vi "ProcessPulses_v1k.vi"() -> ()   [LabVIEW 2013]
uses:
  <vilib>/Utility/error.llb/whitespace.ctl
  <vilib>/Analysis/baseanly.llb/Mean (DBL).vi
  <vilib>/Utility/file.llb/Read From Spreadsheet File (DBL).vi
  <vilib>/Utility/file.llb/Read From Spreadsheet File (string).vi
  <vilib>/Analysis/NI_AALBase.lvlib
panel:
  in  "Stop All":bool
  in  "Tab Control":enum32{"Isotope Results", "Summary Table"}(tab)
  in  "AddedToSummary?":bool
  in  "CalculationDone?":bool
  in  "FileLoaded?":bool
  in  "FileSuffix":string=".str.csv"
  in  "AnalysisID":u32 format="%04.0f"
  in  "PulseDataFilesDirectory":path
  in  "FileToLoadExists?":bool
  in  "ExpressLoad":bool
  in  "FileToLoad":path
  in  "MessageOut":string
  out "Cycle Data":dbl[][](array[numeric])
  out "CycleData":string[](array[string])
  out "Pulse Data":dbl[][](array[numeric])
  out "Results array loaded from file:":path
  out "low":dbl format="%.2f"
  out "high":dbl format="%.2f"
  out "width":dbl format="%.2f"
  in  "Confidence Level":dbl=95.0 format="%#.2f"
  in  "Open a saved spreadsheet?":bool
  out "rel mean diff Press vs Ref":dbl format="%.2f"
  out "Ratios, Sam/Ref":dbl[][](array[numeric]) format="%10.2f"
  out "diff MR CH4 vs Ref":dbl format="%.2f"
  in  "Line to clear from array:":i32
  in  "Clear this line?":bool
  out "Results array saved to file:":path
  in  "Save array to spreadsheet? (NOT FUNCTIONAL YET)":bool
  in  "Last Cycle to Use":i32=16
  in  "First Cycle to Use":dbl=1.0
  out "# of Comparisons":i32
  in  "Calculate Now?":bool
  out "Mean and SD Ratios":dbl[][](array[numeric]) format="%10.2f"
  in  "Which Order?":enum16{"No Calculation", "Ref-Sam", "Sam-Ref"}(ring)=enum."Sam-Ref" caption="Calculate using which sam/ref order?"
  out "diff Press vs Ref":dbl format="%.2f"
  in  "Method":T1(ring)
  in  "PulseData":string[](array[string])
  in  "AutoScroll?":bool=TRUE
  out "tStampToAppend":string
  out "SummaryTableTimestamps":string[](array[string]) caption="ISO-8601 Timestamp"
  in  "Save Table to File?":bool
  in  "Clear whole table?":bool
  in  "SummaryTableFilePath":path
  out "FilenameToBeAdded":string
  out "Array to Append":dbl[](array[numeric])
  in  "Line to clear from Summary":i32
  in  "Clear line from Summary?":bool
  out "SummaryTableLineNumber":i32[](array[numeric]) caption="Line #"
  out "SummaryTableFilenames":string[](array[string]) caption="STR Filename"
  out "SummaryTable":string[](array[string])
  out "Summary Table":dbl[][](array[numeric])
  in  "Add to Summary?":bool
  # "EXPRESS Keyboard Shortcuts:   [F1] Increment Filename,  [F2] Load File,  [F3] Calculate,  [F4] Add Results to Summary Table,  [F5] Change focus to Isotope Results Tab"
  # "(zero-indexed)"
  # "(pop up dialog will open)"
  # "(this menu only used for S-R or R-S \ncomparison method)"
  # "(pop up dialog will open)"
  # "Q/Qref - 1"
  # "Q/Qref - 1"
  # "d13, dD, d13D, D13D\nstdev's"
  # "%"
  # "%"
  # "%"
  # "%"
  # "(zero-indexed)"
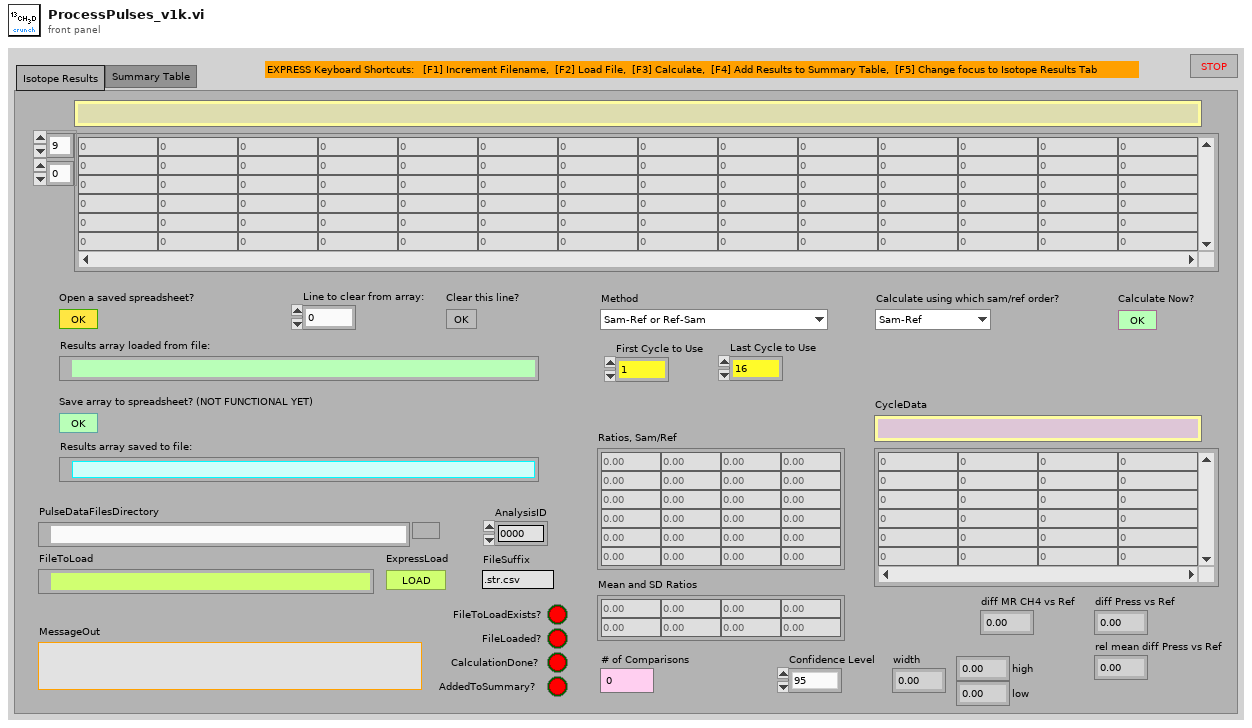
[diagram p1: front panel]
types:
  T1 = enum16{"Sam-Ref or Ref-Sam", "Recycle (Ref-Sam-Ref)"}
  T2 = typedef "whitespace.ctl" = u16
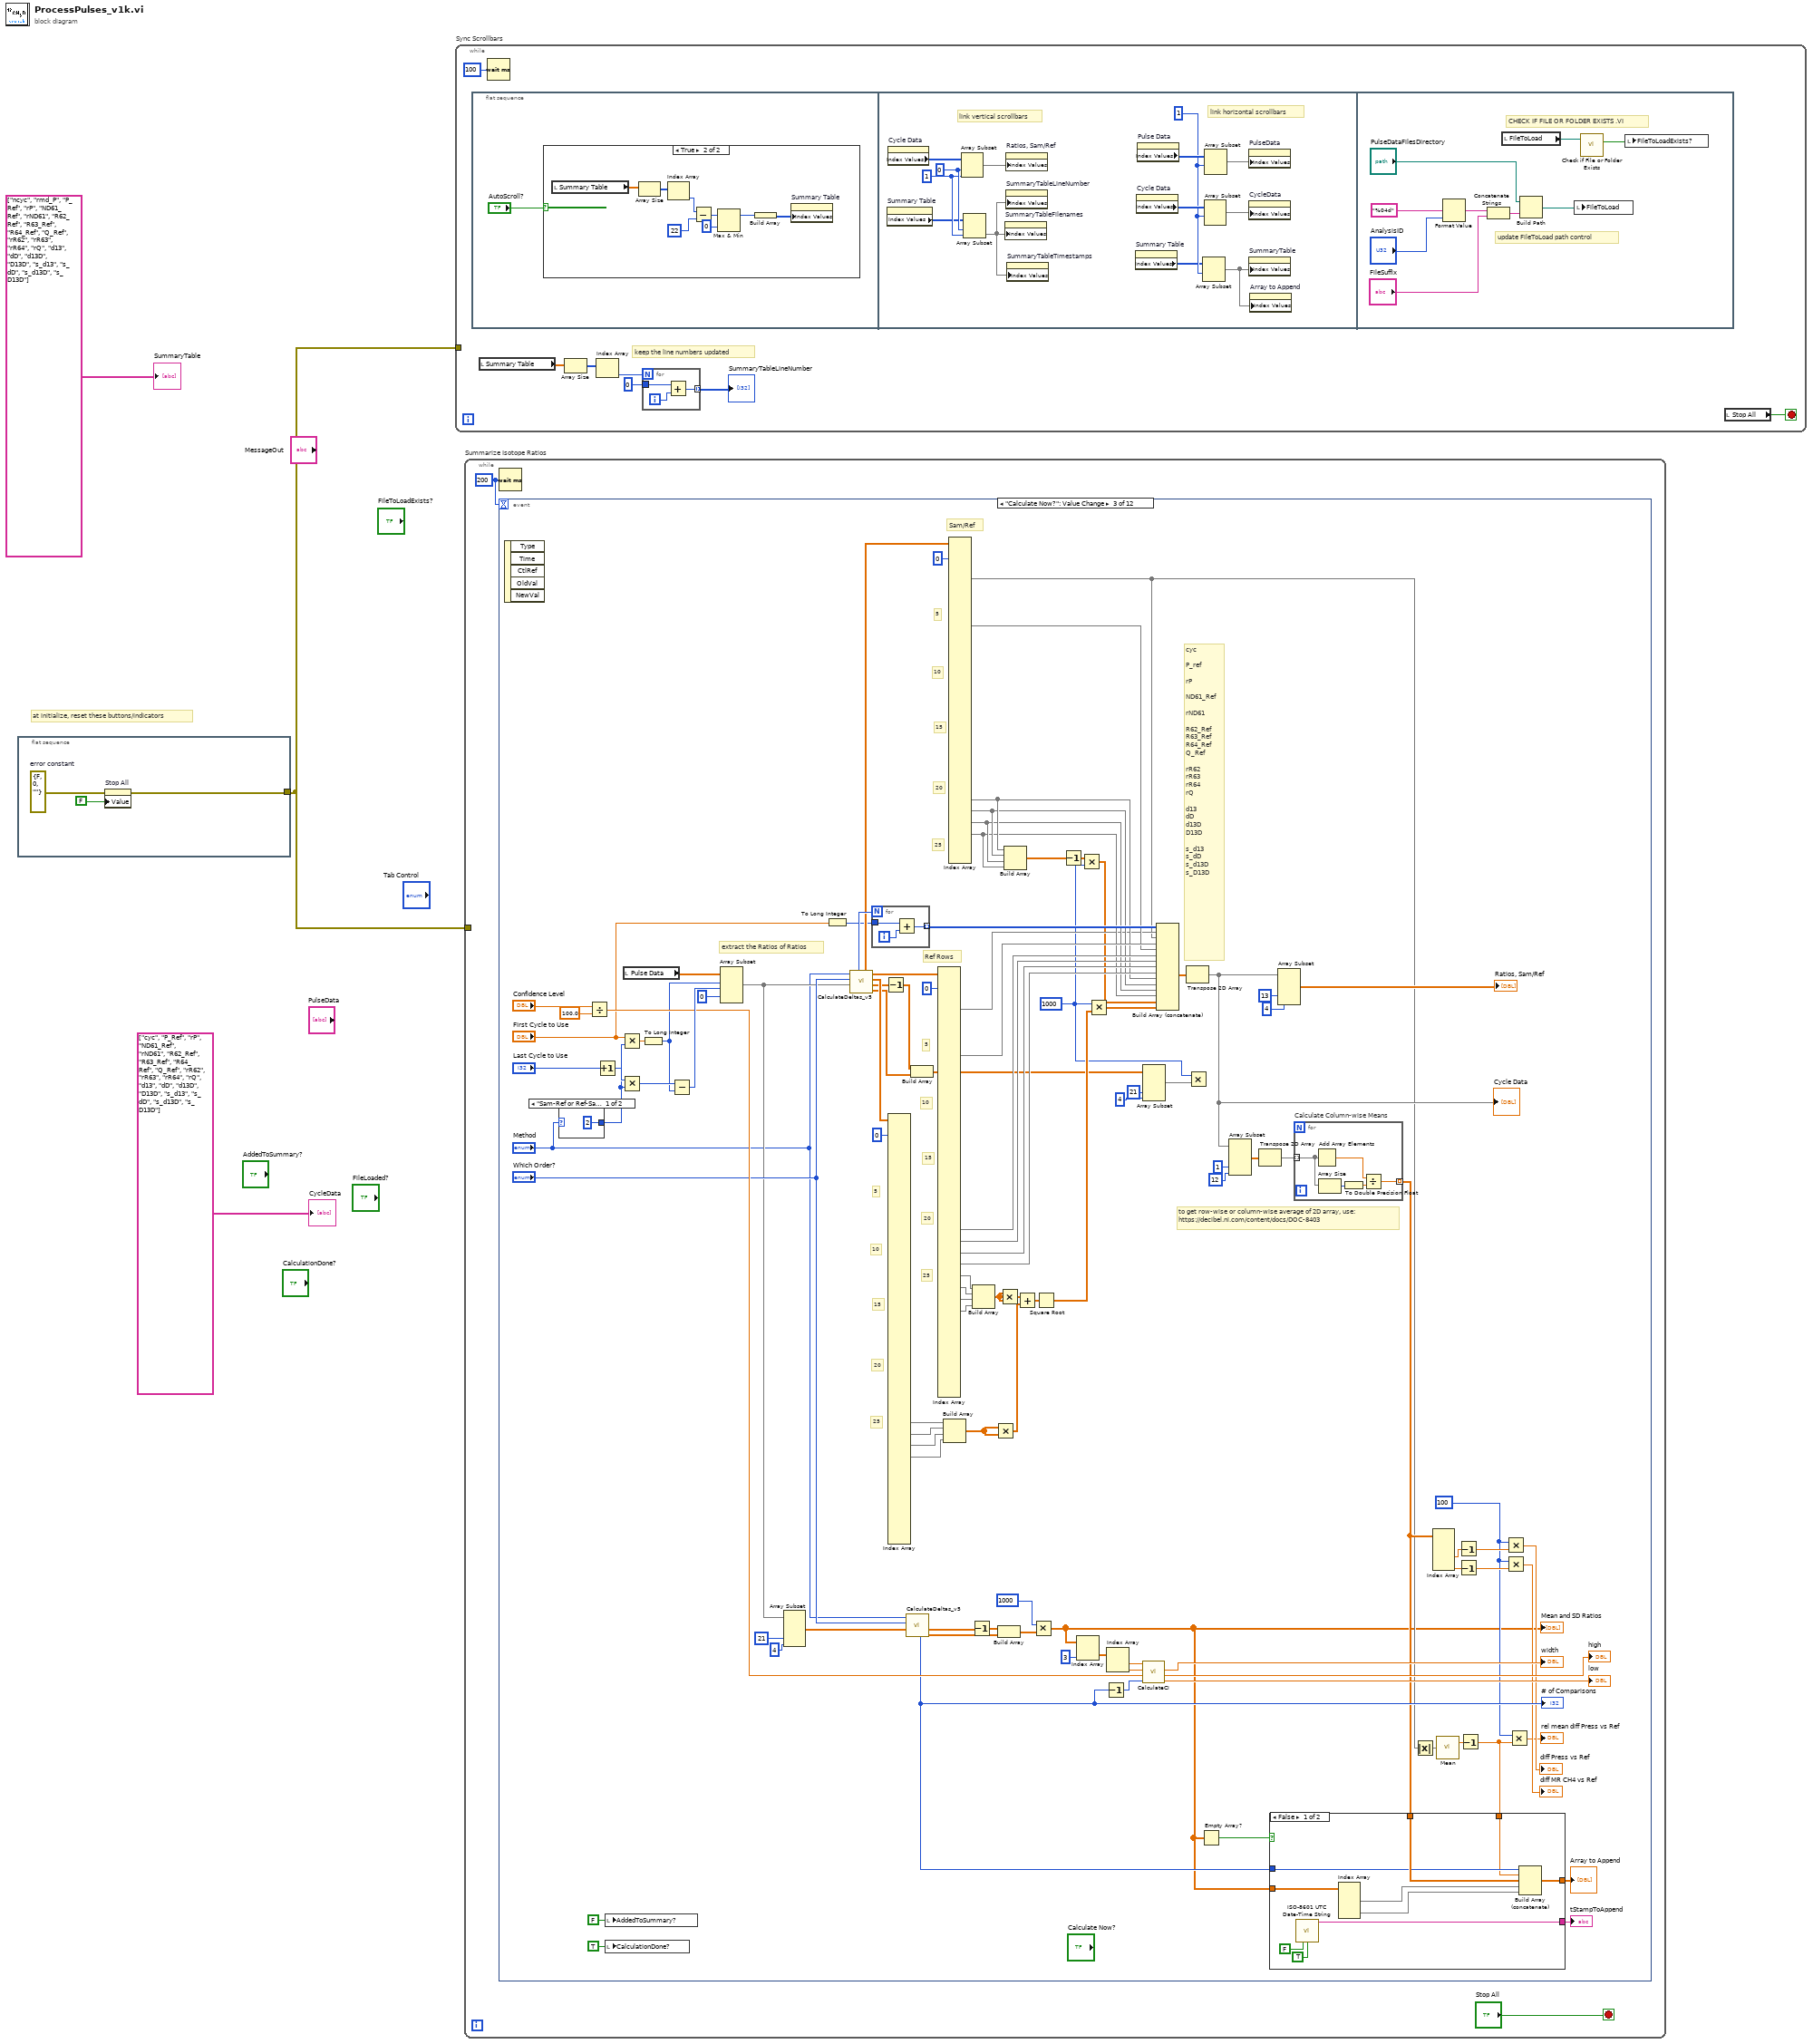
[diagram p0: block diagram]
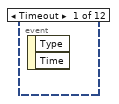
[diagram p3: hidden frame]
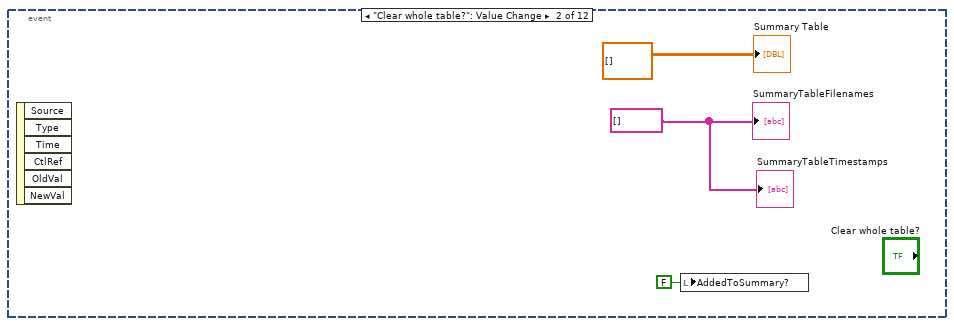
[diagram p4: hidden frame]
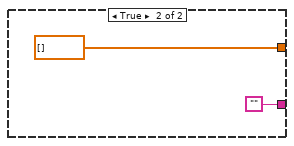
[diagram p5: hidden frame]
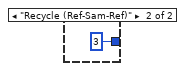
[diagram p6: hidden frame]
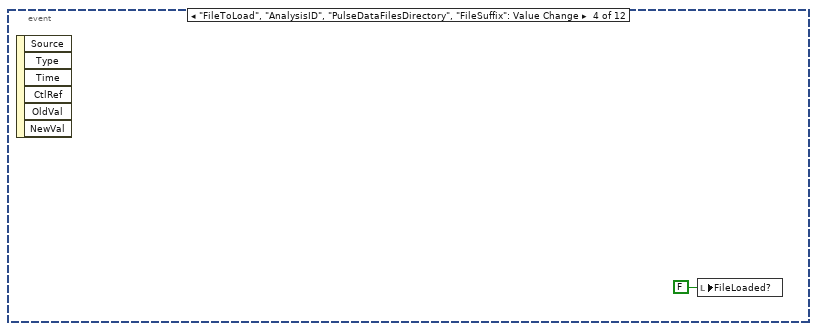
[diagram p7: hidden frame]
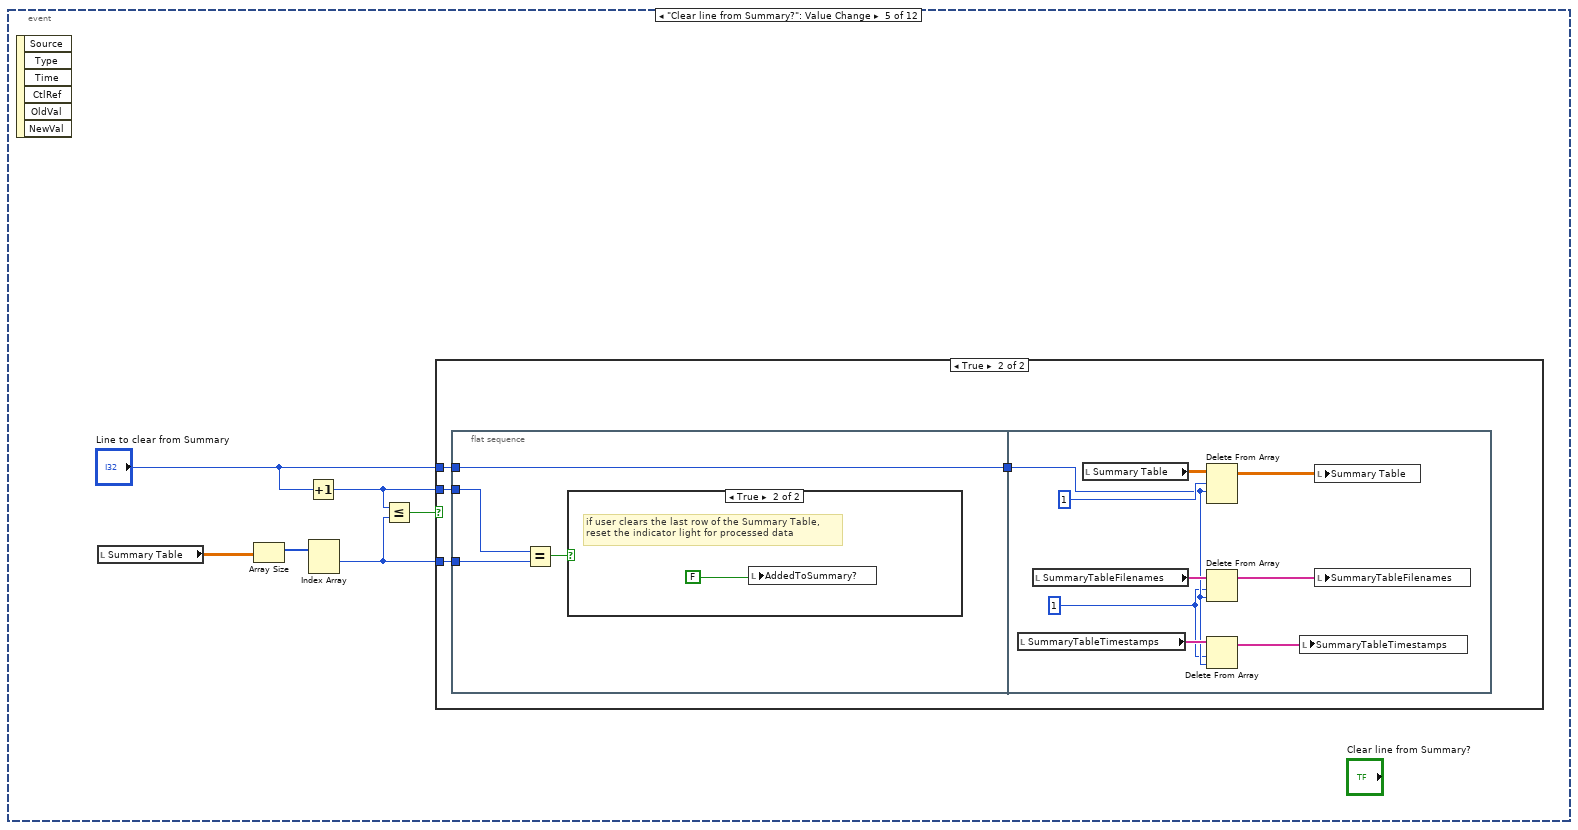
[diagram p8: hidden frame]
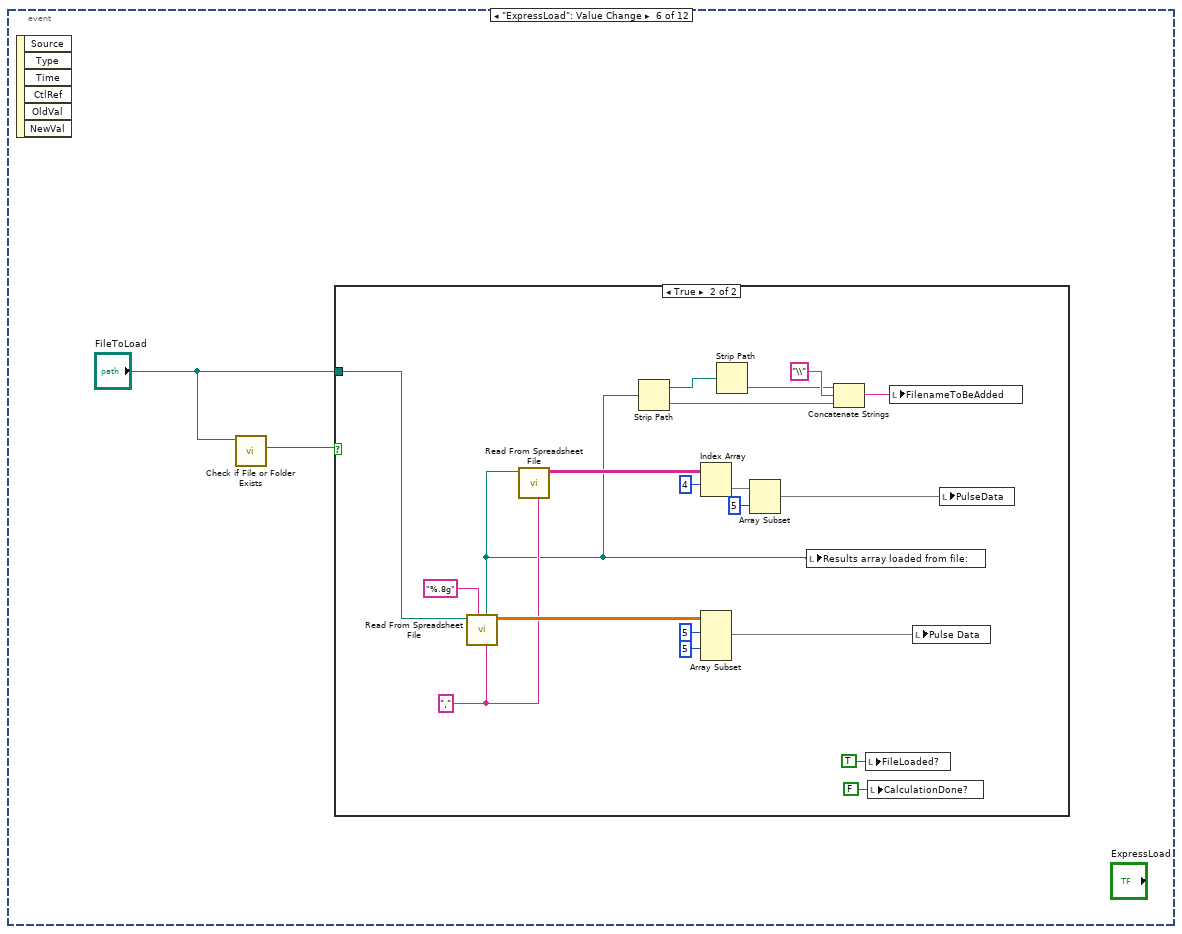
[diagram p11: hidden frame]
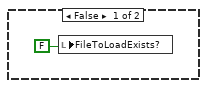
[diagram p12: hidden frame]
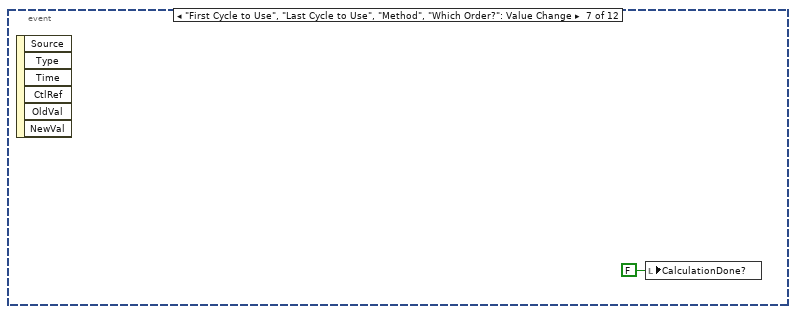
[diagram p13: hidden frame]
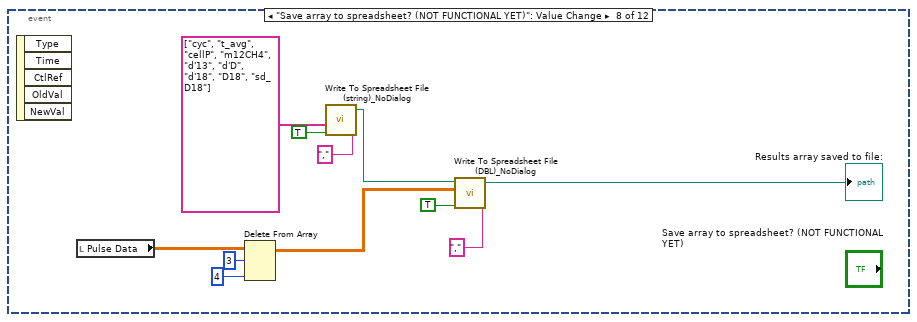
[diagram p14: hidden frame]
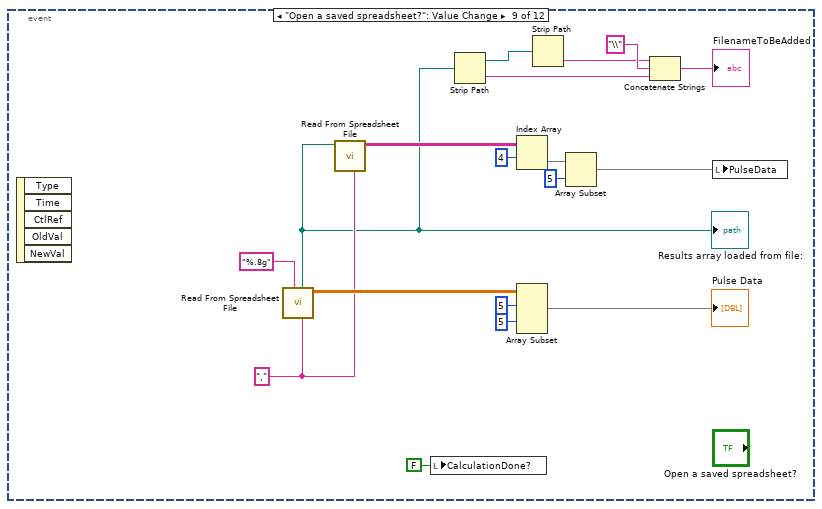
[diagram p15: hidden frame]
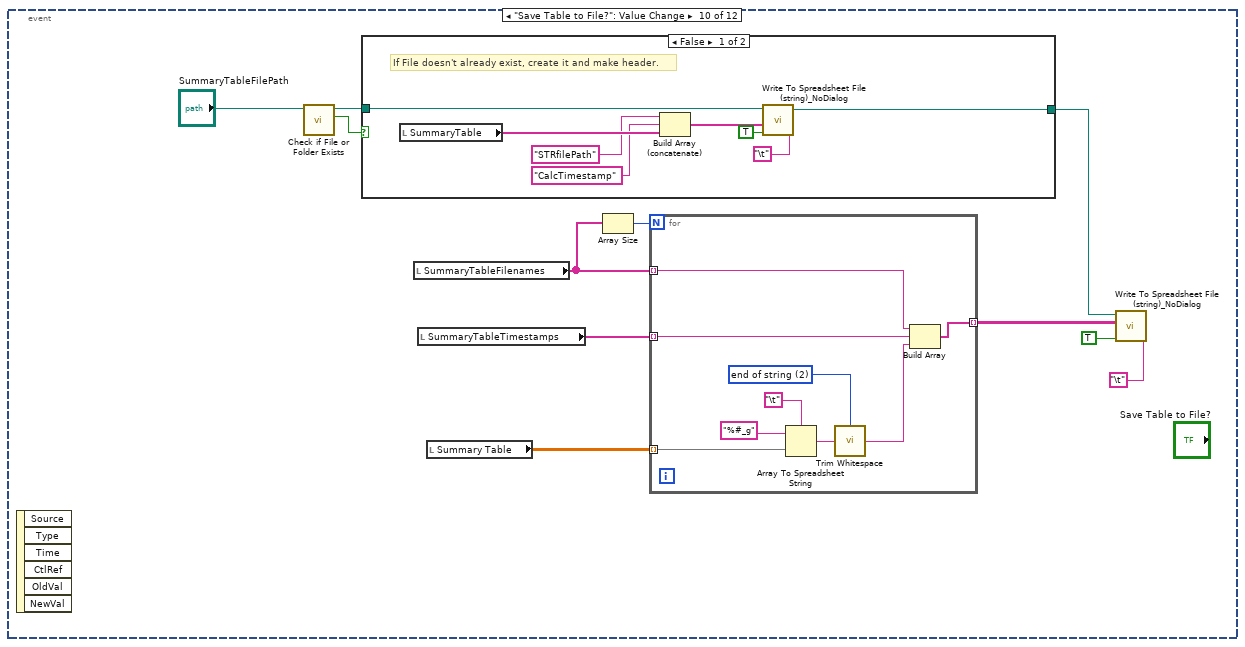
[diagram p16: hidden frame]
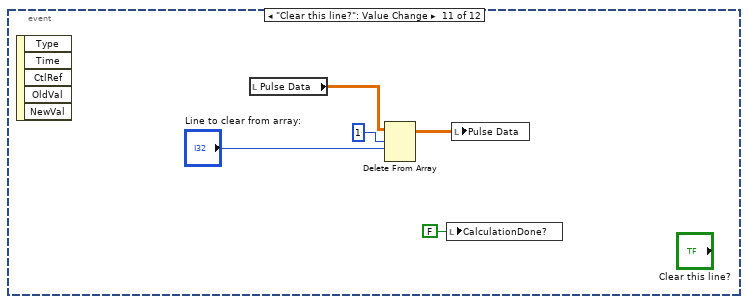
[diagram p18: hidden frame]
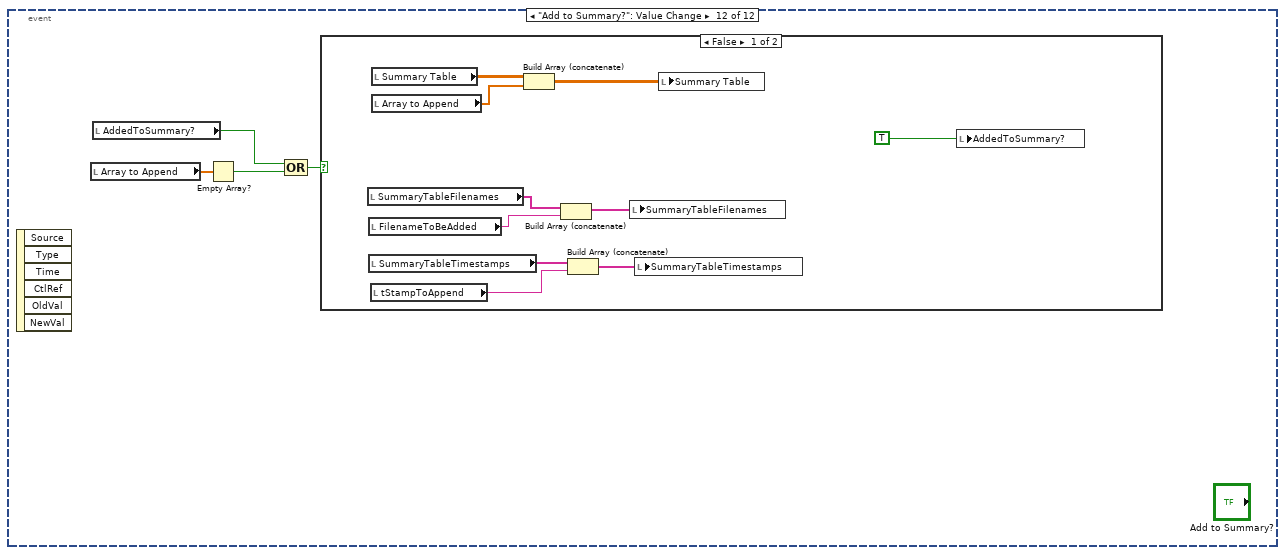
[diagram p19: hidden frame]
diagram:
  # "at initialize, reset these buttons/indicators"
  n1 = flat-sequence {
    tunnel: [w4] -> w3
    frame #0 {
      w5 = errorcluster {"status"=FALSE, "code"=0, "source"=""}  # error constant
      n2 = property on="Stop All" class="Bool (strict)"(error in=w5, "Value"=FALSE) -> (error out=w4:errorcluster)  [unwired: 1 in, 1 out]
    }
  }
  n3 = while "Sync Scrollbars" {
    tunnel: w3 -> [_]
    stop <- w13 stop-if-true
    # "keep the line numbers updated"
    n4 = flat-sequence {
      frame #0 {
        n5 = case shown="True" "AutoScroll?" {
          frame False {
          }
          frame True {
            n6 = local read "Summary Table"() -> (w15:dbl[][])
            n7 = Array Size(array=w15) -> (size(s)=w16:i32[])
            n8 = Index Array(array=w16) -> (element=w17:i32)  [unwired: 1 in]
            n9 = Subtract(x=w17, y=u32 22) -> (x-y=w20:u32)
            n10 = Max & Min(x=w20, y=u32 0) -> (max(x,y)=w19:u32)  [unwired: 1 out]
            n11 = Build Array(w19) -> (w22:u32[])
            n12 = property on="Summary Table" class="Arr (strict)"("Index Values"=w22) -> ()  [unwired: 2 in, 2 out]
          }
        }
      }
      frame #1 {
        w27 = 1 ("length")
        w28 = 0 ("index")
        w29 = 1 ("index")
        # "link vertical scrollbars"
        # "link horizontal scrollbars"
        n13 = property on="Summary Table" class="Arr (strict)"() -> ("Index Values"=w26:u32[])  [unwired: 2 in, 2 out]
        n14 = property on="Cycle Data" class="Arr (strict)"() -> ("Index Values"=w31:u32[])  [unwired: 2 in, 2 out]
        n15 = Array Subset(array=w31, index=w28, length=w27) -> (w30:u32[])
        n16 = Array Subset(array=w26, index=w28, length=w27) -> (w23:u32[])
        n17 = property on="SummaryTableFilenames" class="Arr (strict)"("Index Values"=w23) -> ()  [unwired: 2 in, 2 out]
        n18 = property on="Ratios, Sam/Ref" class="Arr (strict)"("Index Values"=w30) -> ()  [unwired: 2 in, 2 out]
        n19 = property on="SummaryTableLineNumber" class="Arr (strict)"("Index Values"=w23) -> ()  [unwired: 2 in, 2 out]
        n20 = property on="SummaryTableTimestamps" class="Arr (strict)"("Index Values"=w23) -> ()  [unwired: 2 in, 2 out]
        n21 = property on="Summary Table" class="Arr (strict)"() -> ("Index Values"=w25:u32[])  [unwired: 2 in, 2 out]
        n22 = property on="Cycle Data" class="Arr (strict)"() -> ("Index Values"=w33:u32[])  [unwired: 2 in, 2 out]
        n23 = property on="Pulse Data" class="Arr (strict)"() -> ("Index Values"=w35:u32[])  [unwired: 2 in, 2 out]
        n24 = Array Subset(array=w25, index=w29) -> (w24:u32[])  [unwired: 1 in]
        n25 = Array Subset(array=w33, index=w29) -> (w32:u32[])  [unwired: 1 in]
        n26 = Array Subset(array=w35, index=w29) -> (w34:u32[])  [unwired: 1 in]
        n27 = property on="PulseData" class="Arr (strict)"("Index Values"=w34) -> ()  [unwired: 2 in, 2 out]
        n28 = property on="CycleData" class="Arr (strict)"("Index Values"=w32) -> ()  [unwired: 2 in, 2 out]
        n29 = property on="SummaryTable" class="Arr (strict)"("Index Values"=w24) -> ()  [unwired: 2 in, 2 out]
        n30 = property on="Array to Append" class="Arr (strict)"("Index Values"=w24) -> ()  [unwired: 2 in, 2 out]
      }
      frame #2 {
        # "CHECK IF FILE OR FOLDER EXISTS .VI"
        # "update FileToLoad path control"
        n31 = Format Value(format string="%04d", value (0)="AnalysisID") -> (output string=w40:string)  [unwired: 1 in]
        n32 = Concatenate Strings(w40, "FileSuffix") -> (w39:string)
        n33 = local read "FileToLoad"() -> (w37:path)
        n34 = Build Path(base path="PulseDataFilesDirectory", name or relative path=w39) -> (appended path=w42:path)
        n35 = local write "FileToLoad"(w42) -> ()
        n36 = call <vilib>:"Check if File or Folder Exists.vi"("path"=w37) -> ("file or folder exists?"=w36:bool)  [unwired: 8 in, 2 out]
        n37 = local write "FileToLoadExists?"(w36) -> ()
      }
    }
    n38 = local read "Summary Table"() -> (w9:dbl[][])
    n39 = Wait (ms)(milliseconds to wait=u32 100) -> ()  [unwired: 1 out]
    n40 = Array Size(array=w9) -> (size(s)=w8:i32[])
    n41 = Index Array(array=w8) -> (element=w7:i32)  [unwired: 1 in]
    n42 = for {
      N: w7 -> [_]
      tunnel: [w46] -> w11 mode=indexing
      tunnel: 0 -> [w45]
      i -> [w47]
      n43 = Add(x=w45, y=w47) -> (x+y=w46:i32)
    }
    "SummaryTableLineNumber" <- w11
    n44 = local read "Stop All"() -> (w13:bool)
  }
  n45 = while "Summarize Isotope Ratios" {
    tunnel: w3 -> [_]
    stop <- "Stop All" stop-if-true
    w48 = u32 200 ("milliseconds to wait")
    n46 = Wait (ms)(milliseconds to wait=w48) -> ()  [unwired: 1 out]
    n47 = event shown="[2] \"Calculate Now?\": Value Change" {
      selector: _ -> [_ _ _ _ _ _ _ _ _ _ _ _]
      dyn-events: _ -> [_ _ _ _ _ _ _ _ _ _ _ _]
      timeout: w48 -> [_ _ _ _ _ _ _ _ _ _ _ _]
      event Timeout {
        n48 = event-data() -> ()  [unwired: 1 in, 2 out]
      }
      event "Clear whole table?": Value Change {
        w50 = string[] []
        n49 = event-data() -> ()  [unwired: 1 in, 6 out]
        n50 = local write "AddedToSummary?"(FALSE ("AddedToSummary?")) -> ()
        "Summary Table" <- dbl[][] []
        "SummaryTableFilenames" <- w50
        "SummaryTableTimestamps" <- w50
      }
      event "Calculate Now?": Value Change {
        w61 = 100
        w83 = 1000
        # "to get row-wise or column-wise average of 2D array, use: \nhttps://decibel.ni.com/content/docs/DOC-8403"
        # "25"
        # "20"
        # "15"
        # "10"
        # "5"
        # "25"
        # "20"
        # "15"
        # "10"
        # "5"
        # "25"
        # "20"
        # "15"
        # "10"
        # "5"
        # "Sam/Ref"
        # "Ref Rows"
        # "cyc\n\nP_ref\n\nrP\n\nND61_Ref\n\nrND61\n\nR62_Ref\nR63_Ref\nR64_Ref\nQ_Ref\n\nrR62\nrR63\nrR64\nrQ\n\nd13\ndD\nd13D\nD13D\n\ns_d13\ns_dD\ns_d13D\ns_D13D"
        # "extract the Ratios of Ratios"
        n51 = event-data() -> ()  [unwired: 1 in, 5 out]
        n52 = case shown="\"Sam-Ref or Ref-Sam\", Default" "Method" {
          tunnel: [2 3] -> w151
          frame "Sam-Ref or Ref-Sam", Default {
          }
          frame "Recycle (Ref-Sam-Ref)" {
          }
        }
        n53 = Divide(x="Confidence Level", y=100.0) -> (x/y=w144:dbl)
        n54 = Increment(x="Last Cycle to Use") -> (x+1=w154:i32)
        n55 = local write "AddedToSummary?"(FALSE ("AddedToSummary?")) -> ()
        n56 = local write "CalculationDone?"(TRUE ("CalculationDone?")) -> ()
        n57 = Multiply(x="First Cycle to Use", y=w151) -> (x*y=w153:dbl)
        n58 = Multiply(x=w154, y=w151) -> (x*y=w152:i32)
        n59 = local read "Pulse Data"() -> (w156:dbl[][])
        n60 = To Long Integer(number=w153) -> (32bit integer=w126:i32)
        n61 = Subtract(x=w152, y=w126) -> (x-y=w155:i32)
        n62 = Array Subset "Array Subset"(array=w156, index (row)=w126, length (row)=w155, index (col)=0 ("index")) -> (w133:dbl[][])  [unwired: 1 in]
        n63 = Array Subset "Array Subset"(array=w133, index (col)=21 ("index"), length (col)=4 ("length")) -> (w137:dbl[][])  [unwired: 2 in]
        n64 = To Long Integer(number="First Cycle to Use") -> (32bit integer=w105:i32)
        n65 = call "CalculateDeltas_v5.vi"("Method"="Method", "Which Order?"="Which Order?", "Input 2D Numeric Array"=w133) -> ("Array - Ratio Sam/Ref"=w130:dbl[][], "Number of Comparisons"=w135:i32, "Array - Ref Rows"=w132:dbl[][], "Array - Sample Rows"=w91:dbl[][], "Column-wise Mean of Ratios"=w86:dbl[], "Column-wise STDEVs of Ratios"=w90:dbl[])  [unwired: 1 in]
        n66 = for {
          N: w135 -> [_]
          tunnel: w105 -> [w179]
          tunnel: [w177] -> w134 mode=indexing
          i -> [w178]
          n67 = Add(x=w179, y=w178) -> (x+y=w177:i32)
        }
        n68 = Decrement(x=w86) -> (x-1=w85:dbl[])
        n69 = Index Array(array=w91, index (col) #1=0 ("disabled index (col)")) -> (element #26=w120:dbl[], element #27=w119:dbl[], element #28=w118:dbl[], element #29=w117:dbl[])  [unwired: 71 in, 32 out]
        n70 = call "CalculateDeltas_v5.vi"("Method"="Method", "Which Order?"="Which Order?", "Input 2D Numeric Array"=w137) -> ("Number of Comparisons"=w78:i32, "Column-wise Mean of Ratios"=w82:dbl[], "Column-wise STDEVs of Ratios"=w158:dbl[])  [unwired: 1 in, 3 out]
        "# of Comparisons" <- w78
        n71 = Build Array(w85, w90) -> (w89:dbl[][])
        n72 = Index Array(array=w132, index (col) #1=0 ("disabled index (col)")) -> (element #3=w103:dbl[], element #7=w128:dbl[], element #22=w125:dbl[], element #23=w124:dbl[], element #24=w123:dbl[], element #25=w122:dbl[], element #26=w116:dbl[], element #27=w115:dbl[], element #28=w114:dbl[], element #29=w113:dbl[])  [unwired: 71 in, 26 out]
        n73 = Build Array(w120, w119, w118, w117) -> (w100:dbl[][])
        n74 = Index Array(array=w130, index (col) #1=0 ("disabled index (col)")) -> (element #3=w65:dbl[], element #7=w127:dbl[], element #22=w110:dbl[], element #23=w109:dbl[], element #24=w108:dbl[], element #25=w107:dbl[])  [unwired: 53 in, 21 out]
        n75 = Decrement(x=w82) -> (x-1=w81:dbl[])
        n76 = Build Array(w116, w115, w114, w113) -> (w101:dbl[][])
        n77 = Multiply(x=w100, y=w100) -> (x*y=w112:dbl[][])
        n78 = Build Array "Build Array"(w81, w158) -> (w80:dbl[][])
        n79 = Multiply(x=w101, y=w101) -> (x*y=w102:dbl[][])
        n80 = Build Array(w110, w109, w108, w107) -> (w98:dbl[][])
        n81 = Add(x=w102, y=w112) -> (x+y=w111:dbl[][])
        n82 = Multiply(x=1000, y=w80) -> (x*y=w60:dbl[][])
        "Mean and SD Ratios" <- w60
        n83 = Square Root(x=w111) -> (sqrt(x)=w97:dbl[][])
        n84 = Decrement(x=w98) -> (x-1=w99:dbl[][])
        n85 = Index Array(array=w60, index (col)=3 ("disabled index (col)")) -> (element=w149:dbl[])  [unwired: 1 in]
        n86 = Multiply(x=w99, y=w83) -> (x*y=w96:dbl[][])
        n87 = Multiply(x=w83, y=w97) -> (x*y=w95:dbl[][])
        n88 = Decrement(x=w78) -> (x-1=w140:i32)
        n89 = Index Array(array=w149) -> (element #1=w148:dbl, element #2=w147:dbl)  [unwired: 2 in]
        n90 = call "CalculateCI.vi"("k degrees of freedom (n-1)"=w140, "Confidence Level"=w144, "Standard Deviation"=w147, "Mean"=w148) -> ("low"=→"low":dbl, "high"=→"high":dbl, "Width"=→"width":dbl)  [unwired: 5 in]
        n91 = Array Subset(array=w89, index (col)=21 ("index"), length (col)=4 ("length")) -> (w84:dbl[][])  [unwired: 2 in]
        n92 = Build Array (concatenate)(w134, w103, w65, w128, w127, w125, w124, w123, w122, w110, w109, w108, w107, w96, w95) -> (w106:dbl[][])
        n93 = Transpose 2D Array(2D array=w106) -> (transposed array=w76:dbl[][])
        "Cycle Data" <- w76
        n94 = Multiply(x=w83, y=w84) -> ()  [unwired: 1 out]
        n95 = Empty Array?(array=w60) -> (empty?=w59:bool)
        n96 = Array Subset "Array Subset"(array=w76, index (col)=1 ("index"), length (col)=12 ("length")) -> (w73:dbl[][])  [unwired: 2 in]
        n97 = Transpose 2D Array(2D array=w73) -> (transposed array=w72:dbl[][])
        n98 = Array Subset(array=w76, index (col)=13 ("index"), length (col)=4 ("length")) -> (→"Ratios, Sam/Ref":dbl[][])  [unwired: 2 in]
        n99 = for "Calculate Column-wise Means" {
          tunnel: w72 -> [w174] mode=indexing
          tunnel: [w175] -> w71 mode=indexing
          n100 = Add Array Elements(numeric array=w174) -> (sum=w176:dbl)
          n101 = Array Size(array=w174) -> (size(s)=w173:i32)
          n102 = To Double Precision Float(number=w173) -> (double precision float=w172:dbl)
          n103 = Divide(x=w176, y=w172) -> (x/y=w175:dbl)
        }
        n104 = Absolute Value(x=w65) -> (abs(x)=w63:dbl[])
        n105 = Index Array(array=w71) -> (element #3=w67:dbl, element #5=w70:dbl)  [unwired: 5 in, 3 out]
        n106 = call-poly <vilib>:"Mean.vi"("X"=w63) -> ("mean"=w64:dbl)  [unwired: 1 out]
        n107 = Decrement(x=w67) -> (x-1=w66:dbl)
        n108 = Decrement(x=w70) -> (x-1=w69:dbl)
        n109 = Decrement(x=w64) -> (x-1=w53:dbl)
        n110 = case shown="False" w59 {
          tunnel: w78 -> [w164 _]
          tunnel: [w169 dbl[] []] -> w77
          tunnel: w71 -> [w166 _]
          tunnel: w60 -> [w165 _]
          tunnel: [w161 ""] -> w54
          tunnel: w53 -> [w160 _]
          frame False {
            n111 = call "ISO-8601 UTC Date-Time String.vi"("Include TZ? (T)"=FALSE, "Basic? (F)"=TRUE) -> ("8601 Date/Time String"=w161:string)  [unwired: 11 in, 2 out]
            n112 = Index Array "Index Array"(array=w165) -> (element #1=w167:dbl[], element #2=w168:dbl[])  [unwired: 4 in]
            n113 = Build Array (concatenate)(w164, w160, w166, w167, w168) -> (w169:dbl[])
          }
          frame True {
          }
        }
        "Array to Append" <- w77
        "tStampToAppend" <- w54
        n114 = Multiply(x=w61, y=w66) -> (x*y=→"diff Press vs Ref":dbl)
        n115 = Multiply(x=w61, y=w69) -> (x*y=→"diff MR CH4 vs Ref":dbl)
        n116 = Multiply(x=w61, y=w53) -> (x*y=→"rel mean diff Press vs Ref":dbl)
      }
      event "FileToLoad", "AnalysisID", "PulseDataFilesDirectory", "FileSuffix": Value Change {
        n117 = event-data() -> ()  [unwired: 1 in, 6 out]
        n118 = local write "FileLoaded?"(FALSE ("FileLoaded?")) -> ()
      }
      event "Clear line from Summary?": Value Change {
        n119 = event-data() -> ()  [unwired: 1 in, 6 out]
        n120 = local read "Summary Table"() -> (w187:dbl[][])
        n121 = Array Size(array=w187) -> (size(s)=w186:i32[])
        n122 = Increment(x="Line to clear from Summary") -> (x+1=w183:i32)
        n123 = Index Array(array=w186) -> (element #1=w185:i32)  [unwired: 2 in, 1 out]
        n124 = Less Or Equal?(x=w183, y=w185) -> (x <= y?=w188:bool)
        n125 = case shown="True" w188 {
          tunnel: "Line to clear from Summary" -> [_ w191]
          tunnel: w185 -> [_ w192]
          tunnel: w183 -> [_ w189]
          frame False {
            # "do nothing if out of range"
          }
          frame True {
            n126 = flat-sequence {
              tunnel: w192 -> [w195]
              tunnel: w191 -> [w194]
              tunnel: [w194] -> w190
              tunnel: w189 -> [w193]
              tunnel: w190 -> [w200]
              frame #0 {
                n127 = Equal?(x=w193, y=w195) -> (x = y?=w196:bool)
                n128 = case shown="True" w196 {
                  frame False {
                  }
                  frame True {
                    # "if user clears the last row of the Summary Table, \nreset the indicator light for processed data"
                    n129 = local write "AddedToSummary?"(FALSE) -> ()
                  }
                }
              }
              frame #1 {
                w199 = 1 ("length")
                n130 = local read "SummaryTableTimestamps"() -> (w201:string[])
                n131 = local read "SummaryTableFilenames"() -> (w203:string[])
                n132 = local read "Summary Table"() -> (w204:dbl[][])
                n133 = Delete From Array "Delete From Array"(array=w204, length=1, index (row)=w200) -> (array with subset deleted=w205:dbl[][])  [unwired: 1 in, 1 out]
                n134 = Delete From Array "Delete From Array"(array=w203, length=w199, index=w200) -> (array with subset deleted=w202:string[])  [unwired: 1 out]
                n135 = Delete From Array "Delete From Array"(array=w201, length=w199, index=w200) -> (array with subset deleted=w198:string[])  [unwired: 1 out]
                n136 = local write "SummaryTableTimestamps"(w198) -> ()
                n137 = local write "Summary Table"(w205) -> ()
                n138 = local write "SummaryTableFilenames"(w202) -> ()
              }
            }
          }
        }
      }
      event "ExpressLoad": Value Change {
        n139 = event-data() -> ()  [unwired: 1 in, 6 out]
        n140 = call <vilib>:"Check if File or Folder Exists.vi"("path"="FileToLoad") -> ("file or folder exists?"=w208:bool)  [unwired: 8 in, 2 out]
        n141 = case shown="True" w208 {
          tunnel: "FileToLoad" -> [_ w216]
          frame False {
            n142 = local write "FileToLoadExists?"(FALSE) -> ()
          }
          frame True {
            w223 = "," ("delimiter (\\t)")
            n143 = call-poly <vilib>:"Read From Spreadsheet File.vi"("delimiter (\\t)"=w223, "format (%.3f)"="%.8g", "file path (dialog if empty)"=w216) -> ("all rows"=w226:dbl[][], "new file path (Not A Path if cancelled)"=w212:path)  [unwired: 4 in, 3 out]
            n144 = call-poly <vilib>:"Read From Spreadsheet File.vi"("delimiter (\\t)"=w223, "file path (dialog if empty)"=w212) -> ("all rows"=w228:string[][])  [unwired: 5 in, 4 out]
            n145 = Strip Path(path=w212) -> (stripped path=w217:path, name=w220:string)
            n146 = Index Array "Index Array"(array=w228, index (row)=4) -> (element=w222:string[])  [unwired: 1 in]
            n147 = Array Subset "Array Subset"(array=w226, index (row)=5 ("index"), index (col)=5 ("index")) -> (w213:dbl[][])  [unwired: 2 in]
            n148 = Strip Path(path=w217) -> (name=w218:string)  [unwired: 1 out]
            n149 = Array Subset "Array Subset"(array=w222, index=5) -> (w214:string[])  [unwired: 1 in]
            n150 = local write "Results array loaded from file:"(w212) -> ()
            n151 = Concatenate Strings(w218, "\\" ("string"), w220) -> (w215:string)
            n152 = local write "FileLoaded?"(TRUE ("FileLoaded?")) -> ()
            n153 = local write "CalculationDone?"(FALSE ("CalculationDone?")) -> ()
            n154 = local write "FilenameToBeAdded"(w215) -> ()
            n155 = local write "Pulse Data"(w213) -> ()
            n156 = local write "PulseData"(w214) -> ()
          }
        }
      }
      event "First Cycle to Use", "Last Cycle to Use", "Method", "Which Order?": Value Change {
        n157 = event-data() -> ()  [unwired: 1 in, 6 out]
        n158 = local write "CalculationDone?"(FALSE ("CalculationDone?")) -> ()
      }
      event "Save array to spreadsheet? (NOT FUNCTIONAL YET)": Value Change {
        n159 = event-data() -> ()  [unwired: 1 in, 5 out]
        n160 = local read "Pulse Data"() -> (w238:dbl[][])
        n161 = Delete From Array "Delete From Array"(array=w238, length=3, index (col)=4 ("disabled index (col)")) -> (array with subset deleted=w232:dbl[][])  [unwired: 1 in, 1 out]
        n162 = call "Write To Spreadsheet File (string)_NoDialog.vi"("delimiter (\\t)"="," ("delimiter (\\t)"), "append to file? (new file:F)"=TRUE, "1D data"=string[] ["cyc", "t_avg", "cellP", "m12CH4", "d'13", "d'D", "d'18", "D18", "sd_D18"]) -> ("new file path (Not A Path if cancelled)"=w234:path)  [unwired: 5 in]
        n163 = call "Write To Spreadsheet File (DBL)_NoDialog.vi"("delimiter (\\t)"="," ("delimiter (\\t)"), "append to file? (new file:F)"=TRUE, "2D data"=w232, "file path (dialog if empty)"=w234) -> ("new file path (Not A Path if cancelled)"=→"Results array saved to file:":path)  [unwired: 4 in]
      }
      event "Open a saved spreadsheet?": Value Change {
        w252 = "," ("delimiter (\\t)")
        n164 = event-data() -> ()  [unwired: 1 in, 5 out]
        n165 = call-poly <vilib>:"Read From Spreadsheet File.vi"("delimiter (\\t)"=w252, "format (%.3f)"="%.8g") -> ("all rows"=w256:dbl[][], "new file path (Not A Path if cancelled)"=w248:path)  [unwired: 5 in, 3 out]
        "Results array loaded from file:" <- w248
        n166 = call-poly <vilib>:"Read From Spreadsheet File.vi"("delimiter (\\t)"=w252, "file path (dialog if empty)"=w248) -> ("all rows"=w258:string[][])  [unwired: 5 in, 4 out]
        n167 = local write "CalculationDone?"(FALSE ("CalculationDone?")) -> ()
        n168 = Strip Path(path=w248) -> (stripped path=w243:path, name=w246:string)
        n169 = Index Array "Index Array"(array=w258, index (row)=4) -> (element=w251:string[])  [unwired: 1 in]
        n170 = Array Subset "Array Subset"(array=w256, index (row)=5 ("index"), index (col)=5 ("index")) -> (→"Pulse Data":dbl[][])  [unwired: 2 in]
        n171 = Strip Path(path=w243) -> (name=w244:string)  [unwired: 1 out]
        n172 = Array Subset "Array Subset"(array=w251, index=5) -> (w250:string[])  [unwired: 1 in]
        n173 = Concatenate Strings(w244, "\\" ("string"), w246) -> (→"FilenameToBeAdded":string)
        n174 = local write "PulseData"(w250) -> ()
      }
      event "Save Table to File?": Value Change {
        n175 = event-data() -> ()  [unwired: 1 in, 6 out]
        n176 = call <vilib>:"Check if File or Folder Exists.vi"("path"="SummaryTableFilePath") -> ("file or folder exists?"=w265:bool, "dup path"=w266:path)  [unwired: 8 in, 1 out]
        n177 = case shown="False" w265 {
          tunnel: [w287 w288] -> w268
          tunnel: w266 -> [w285 w288]
          frame False {
            # "If File doesn't already exist, create it and make header."
            n178 = local read "SummaryTable"() -> (w282:string[])
            n179 = Build Array (concatenate)("STRfilePath", "CalcTimestamp", w282) -> (w283:string[])
            n180 = call "Write To Spreadsheet File (string)_NoDialog.vi"("delimiter (\\t)"="\t" ("delimiter (\\t)"), "append to file? (new file:F)"=TRUE, "1D data"=w283, "file path (dialog if empty)"=w285) -> ("new file path (Not A Path if cancelled)"=w287:path)  [unwired: 4 in]
          }
          frame True {
            # "If file exists, just append the summary data to the table"
          }
        }
        n181 = local read "SummaryTableFilenames"() -> (w263:string[])
        n182 = local read "SummaryTableTimestamps"() -> (w260:string[])
        n183 = local read "Summary Table"() -> (w264:dbl[][])
        n184 = Array Size(array=w263) -> (size(s)=w262:i32)
        n185 = for {
          N: w262 -> [_]
          tunnel: w263 -> [w276] mode=indexing
          tunnel: w264 -> [w278] mode=indexing
          tunnel: [w275] -> w261 mode=indexing
          tunnel: w260 -> [w271] mode=indexing
          w274 = T2 2 items=["both", "start of string", "end of string"] ("location (both)")
          n186 = Array To Spreadsheet String(delimiter (Tab)="\t", array=w278, 3:"%#_g") -> (spreadsheet string=w273:string)
          n187 = call <vilib>:"Trim Whitespace.vi"("string"=w273, "location (both)"=w274) -> ("trimmed string"=w272:string)
          n188 = Build Array(w276, w271, w272) -> (w275:string[])
        }
        n189 = call "Write To Spreadsheet File (string)_NoDialog.vi"("delimiter (\\t)"="\t", "append to file? (new file:F)"=TRUE, "2D data"=w261, "file path (dialog if empty)"=w268) -> ()  [unwired: 4 in, 1 out]
      }
      event "Clear this line?": Value Change {
        n190 = event-data() -> ()  [unwired: 1 in, 5 out]
        n191 = local read "Pulse Data"() -> (w293:dbl[][])
        n192 = Delete From Array "Delete From Array"(array=w293, length=1, index (row)="Line to clear from array:") -> (array with subset deleted=w290:dbl[][])  [unwired: 1 in, 1 out]
        n193 = local write "CalculationDone?"(FALSE ("CalculationDone?")) -> ()
        n194 = local write "Pulse Data"(w290) -> ()
      }
      event "Add to Summary?": Value Change {
        n195 = event-data() -> ()  [unwired: 1 in, 6 out]
        n196 = local read "Array to Append"() -> (w294:dbl[])
        n197 = local read "AddedToSummary?"() -> (w295:bool)
        n198 = Empty Array?(array=w294) -> (empty?=w296:bool)
        n199 = Compound Arithmetic op=OR(w295, w296) -> (w297:bool)
        n200 = case shown="False" w297 {
          frame False {
            n201 = local read "SummaryTableFilenames"() -> (w304:string[])
            n202 = local read "FilenameToBeAdded"() -> (w303:string)
            n203 = local read "SummaryTableTimestamps"() -> (w300:string[])
            n204 = local read "tStampToAppend"() -> (w299:string)
            n205 = local read "Summary Table"() -> (w307:dbl[][])
            n206 = local read "Array to Append"() -> (w306:dbl[])
            n207 = Build Array (concatenate)(w307, w306) -> (w305:dbl[][])
            n208 = Build Array (concatenate)(w304, w303) -> (w302:string[])
            n209 = Build Array (concatenate)(w300, w299) -> (w298:string[])
            n210 = local write "SummaryTableFilenames"(w302) -> ()
            n211 = local write "SummaryTableTimestamps"(w298) -> ()
            n212 = local write "Summary Table"(w305) -> ()
            n213 = local write "AddedToSummary?"(TRUE) -> ()
          }
          frame True {
          }
        }
      }
    }
  }
  "CycleData" <- string[] ["cyc", "P_Ref", "rP", "ND61_Ref", "rND61", "R62_Ref", "R63_Ref", "R64_Ref", "Q_Ref", "rR62", "rR63", "rR64", "rQ", "d13", "dD", "d13D", "D13D", "s_d13", "s_dD", "s_d13D", "s_D13D"]
  "SummaryTable" <- string[] ["ncyc", "rmd_P", "P_Ref", "rP", "ND61_Ref", "rND61", "R62_Ref", "R63_Ref", "R64_Ref", "Q_Ref", "rR62", "rR63", "rR64", "rQ", "d13", "dD", "d13D", "D13D", "s_d13", "s_dD", "s_d13D", "s_D13D"]
